vi "DSF.Engine.Memory.Index FIFO.Set FIFO Ref.vi"(8 "error in (no error)":errorcluster, 10 "FIFO":refnum<k33>, 11 "Index FIFO in":refnum<class "DSF.Engine.Memory.Index FIFO.lvclass">) -> (0 "error out":errorcluster, 3 "Index FIFO out":refnum<class "DSF.Engine.Memory.Index FIFO.lvclass">)   [LabVIEW 2016, in "DSF.Engine.lvlib" / "DSF.Engine.Memory.Index FIFO.lvclass"]
uses:
  DSF.Engine.Memory.Index FIFO.lvclass
  DSF.Engine.Memory.Index FIFO.lvclass/DSF.Engine.Memory.Index FIFO.ctl
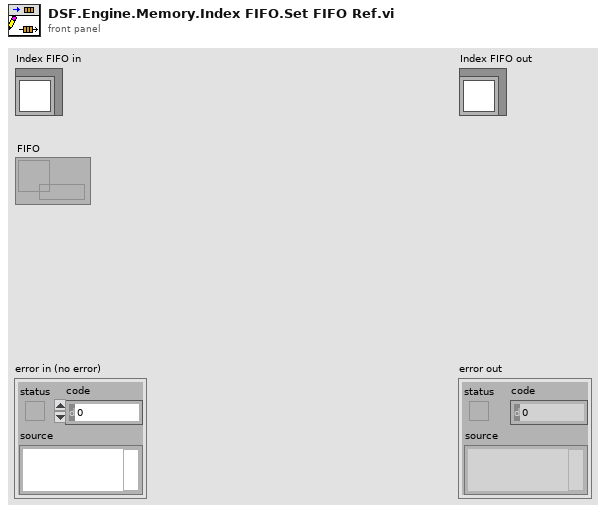
[diagram p1: front panel]
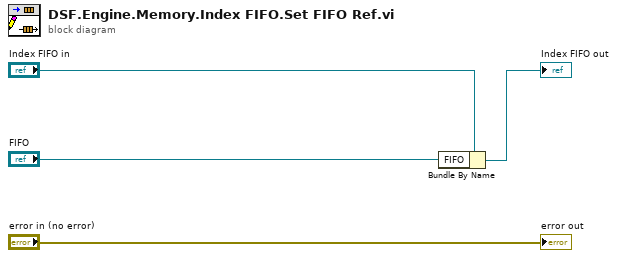
[diagram p0: block diagram]
diagram:
  n1 = Bundle By Name(cluster="Index FIFO in", "FIFO"="FIFO") -> (→"Index FIFO out":refnum<class "DSF.Engine.Memory.Index FIFO.lvclass">)
  "error out" <- "error in (no error)"
